vi "Get Ramp.vi"(8 "error in":errorcluster, 10 "Loop":u8(ring) items=["1", "2", "3", "4"], 11 "VISA in":refnum<visa-resource-name>="tcpip0::192.168.1.5::5000::SOCKET") -> (0 "ErrorOut":errorcluster={"status"=TRUE, "code"=-1073807339, "source"="VISA Read in Cryocon_R/W.vi->Loop_RAMP?.vi"}, 2 "x = y?":bool, 3 "VISA out":refnum<visa-resource-name>="tcpip0::192.168.1.5::5000::SOCKET")   [LabVIEW 2019, in "9T cmag.lvlib"]
uses:
  9T cmag.lvlib
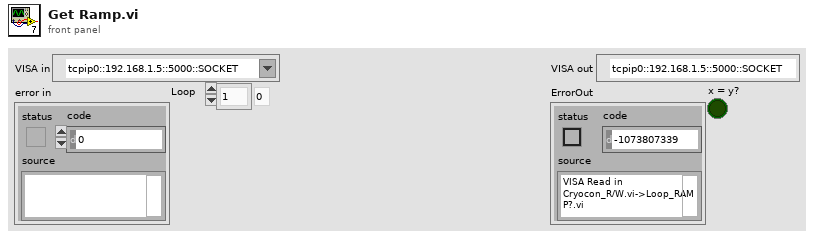
[diagram p1: front panel]
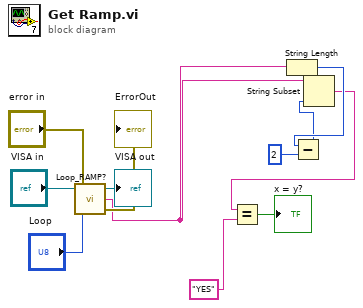
[diagram p0: block diagram]
diagram:
  n1 = call "Loop_RAMP?.vi"("error in"="error in", "Loop"="Loop", "VISA in"="VISA in") -> ("ErrorOut"=→"ErrorOut":errorcluster, "Return"=w5:string, "VISA out"=→"VISA out":refnum<visa-resource-name>)
  n2 = String Length(string=w5) -> (length=w4:i32)
  n3 = Subtract(x=w4, y=2) -> (x-y=w2:i32)
  n4 = String Subset(string=w5, length (rest)=w2) -> (substring=w1:string)  [unwired: 1 in]
  n5 = Equal?(x=w1, y="YES") -> (x = y?=→"x = y?":bool)
